vi "Query S Parameters.vi"(8 "error in (no error)":errorcluster, 10 "Sparameters (string)":string[](array[string]), 11 "VNA-ZNB in":refnum<class "VNA-ZNB.lvclass">) -> (0 "error out":errorcluster, 2 "S Parameters":T1[](array[typedef]), 3 "VNA-ZNB out":refnum<class "VNA-ZNB.lvclass">)   [LabVIEW 2020, in "VNA-ZNB.lvclass"]
doc: "Queryes the S parameter choosen. It can give single parameter or full 2 to 4 port parameters."
uses:
  VNA-ZNB.lvclass
  C:/Sandbox/Git_Sandbox/WiSpry Test Framework source code (LV20)/WiSpry Test Framework/Instruments/Instrument.lvclass
  C:/Sandbox/Git_Sandbox/WiSpry Test Framework source code (LV20)/WiSpry Test Framework/Instruments/Vector Network Analyzer/Vector Network Analyzer.lvclass
  Controls/Sparameter cluster.ctl
  Instrument.lvclass/Instrument.ctl
  Vector Network Analyzer.lvclass/Vector Network Analyzer.ctl
  Instrument.lvclass
  Vector Network Analyzer.lvclass
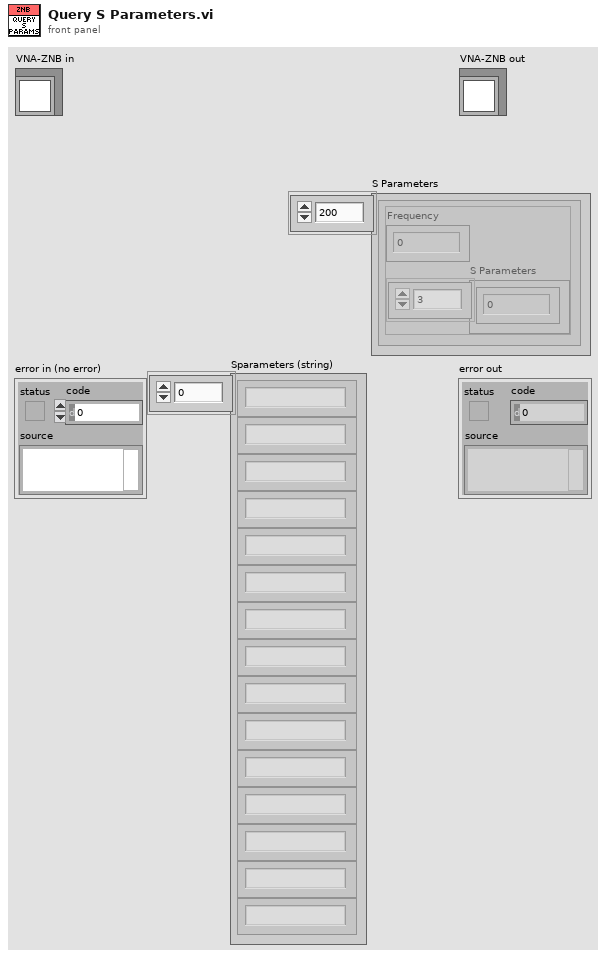
[diagram p1: front panel]
types:
  T1 = typedef "Vector Network Analyzer.lvclass/Sparameter cluster.ctl" = cluster{"Frequency":dbl, "S Parameters":cdb[]}
  T2 = enum16{"big-endian, network order", "native, host order", "little-endian"}
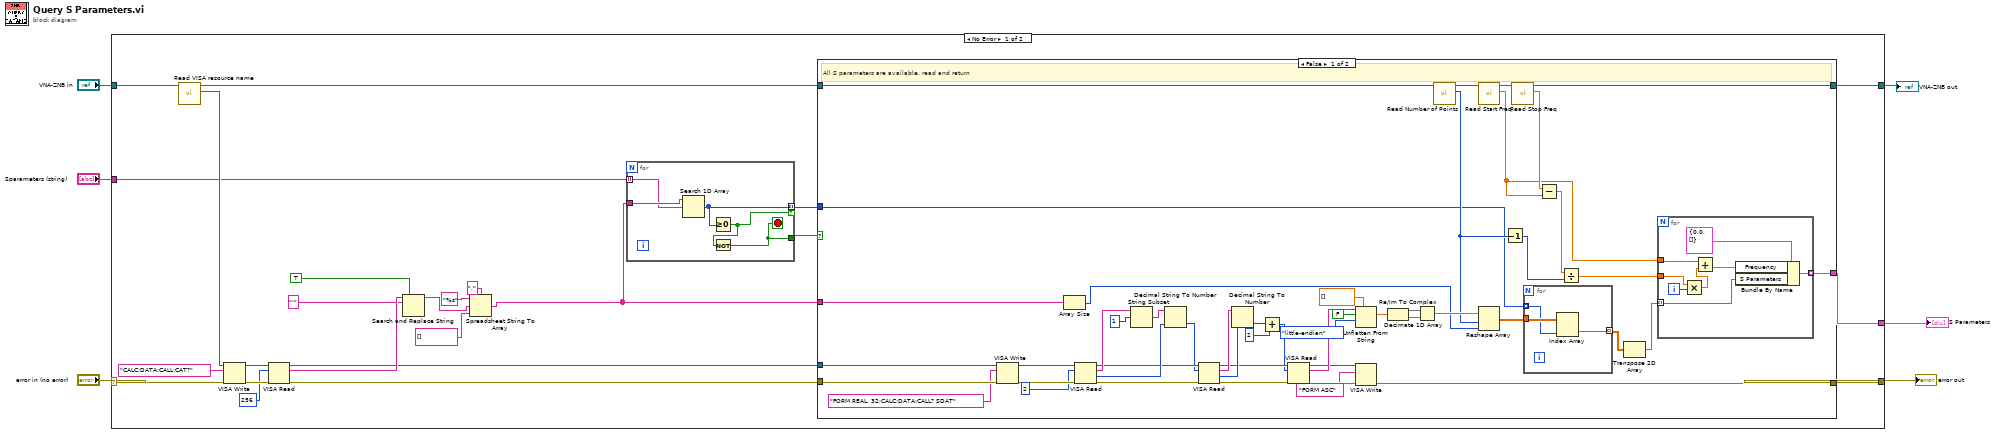
[diagram p0: block diagram]
diagram:
  n1 = case shown="No Error" "error in (no error)" {
    selector: "error in (no error)" -> [w29 w99]
    tunnel: "VNA-ZNB in" -> [w30 w98]
    tunnel: [w13 w98] -> w4
    tunnel: [w8 w99] -> w3
    tunnel: [w12 _] -> w2
    tunnel: "Sparameters (string)" -> [w7 _]
    frame No Error {
      n2 = call "Read VISA resource name.vi"("Instrument in"=w30) -> ("VISA resource name"=w28:refnum<visa-resource-name>, "Instrument out"=w14:refnum<class "VNA-ZNB.lvclass">)  [unwired: 9 in]
      n3 = VISA Write(VISA resource name=w28, write buffer="CALC:DATA:CALL:CAT?", error in (no error)=w29) -> (VISA resource name out=w25:refnum<visa-resource-name>, error out=w26:errorcluster)  [unwired: 1 out]
      n4 = VISA Read(VISA resource name=w25, byte count=u32 256, error in (no error)=w26) -> (VISA resource name out=w15:refnum<visa-resource-name>, read buffer=w23:string, error out=w16:errorcluster)  [unwired: 1 out]
      n5 = Search and Replace String(replace all?=TRUE ("replace all? (F)"), input string=w23, search string="'") -> (result string=w18:string)  [unwired: 5 in, 3 out]
      n6 = Spreadsheet String To Array(delimiter (Tab)=",", format string="%s", spreadsheet string=w18, array type (2D Dbl)=string[] []) -> (array=w11:string[])
      n7 = for {
        tunnel: w7 -> [w96] mode=indexing
        tunnel: w11 -> [w97]
        tunnel: [w95] -> w10 mode=indexing if=w94
        tunnel: [w93] -> w9
        stop <- w93 stop-if-true
        n8 = Search 1D Array(1D array=w97, element=w96) -> (index of element=w95:i32)  [unwired: 1 in]
        n9 = Greater Or Equal To 0?(x=w95) -> (x >= 0?=w94:bool)
        n10 = Not(x=w94) -> (.not. x?=w93:bool)
      }
      n11 = case shown="False" w9 {
        tunnel: w16 -> [w79 w92]
        tunnel: w15 -> [w78 _]
        tunnel: w14 -> [w51 w91]
        tunnel: [w45 w91] -> w13
        tunnel: [w44 _] -> w12
        tunnel: w11 -> [w39 _]
        tunnel: w10 -> [w37 _]
        tunnel: [w31 w92] -> w8
        frame False {
          # "All S parameters are available, read and return"
          n12 = VISA Write(VISA resource name=w78, write buffer="FORM REAL, 32;CALC:DATA:CALL? SDAT", error in (no error)=w79) -> (VISA resource name out=w75:refnum<visa-resource-name>, error out=w76:errorcluster)  [unwired: 1 out]
          n13 = Array Size(array=w39) -> (size(s)=w42:i32)
          n14 = VISA Read(VISA resource name=w75, byte count=u32 2, error in (no error)=w76) -> (VISA resource name out=w68:refnum<visa-resource-name>, read buffer=w71:string, return count=w70:u32, error out=w69:errorcluster)
          n15 = String Subset(string=w71, offset (0)=1) -> (substring=w72:string)  [unwired: 1 in]
          n16 = Decimal String To Number(string=w72, default (0L)=w70) -> (number=w67:u32)  [unwired: 1 in, 1 out]
          n17 = VISA Read(VISA resource name=w68, byte count=w67, error in (no error)=w69) -> (VISA resource name out=w62:refnum<visa-resource-name>, read buffer=w64:string, return count=w63:u32, error out=w60:errorcluster)
          n18 = Decimal String To Number(string=w64, default (0L)=w63) -> (number=w65:u32)  [unwired: 1 in, 1 out]
          n19 = Add(x=w65, y=u32 2) -> (x+y=w61:u32)
          n20 = VISA Read(VISA resource name=w62, byte count=w61, error in (no error)=w60) -> (VISA resource name out=w35:refnum<visa-resource-name>, read buffer=w59:string, error out=w36:errorcluster)  [unwired: 1 out]
          n21 = Unflatten From String(type=sgl[] [], binary string=w59, data includes array or string size? (T)=FALSE, byte order (0:big-endian, network order)=T2."little-endian") -> (value=w55:sgl[])  [unwired: 1 in, 2 out]
          n22 = VISA Write(VISA resource name=w35, write buffer="FORM ASC", error in (no error)=w36) -> (error out=w31:errorcluster)  [unwired: 2 out]
          n23 = Decimate 1D Array(w55) -> (w54:sgl[], w53:sgl[])
          n24 = Re/Im To Complex(1:w53, 2:w54) -> (0:w52:csg[])
          n25 = call "Read Number of Points.vi"("Vector Network Analyzer in"=w51) -> ("Number of Points"=w43:i32, "Vector Network Analyzer out"=w46:refnum<class "VNA-ZNB.lvclass">)  [unwired: 9 in]
          n26 = call "Read Start Freq.vi"("Vector Network Analyzer in"=w46) -> ("Start Freq"=w40:dbl, "Vector Network Analyzer out"=w47:refnum<class "VNA-ZNB.lvclass">)  [unwired: 9 in]
          n27 = Reshape Array(w52, w43, w42) -> (w38:csg[][])
          n28 = Decrement(x=w43) -> (x-1=w41:i32)
          n29 = call "Read Stop Freq.vi"("Vector Network Analyzer in"=w47) -> ("Stop Freq"=w48:dbl, "Vector Network Analyzer out"=w45:refnum<class "VNA-ZNB.lvclass">)  [unwired: 9 in]
          n30 = for {
            tunnel: w38 -> [w82]
            tunnel: w37 -> [w81] mode=indexing
            tunnel: [w80] -> w33 mode=indexing
            n31 = Index Array(array=w82, index (col)=w81) -> (element=w80:csg[])  [unwired: 1 in]
          }
          n32 = Subtract(x=w48, y=w40) -> (x-y=w49:dbl)
          n33 = Divide(x=w49, y=w41) -> (x/y=w50:dbl)
          n34 = Transpose 2D Array(2D array=w33) -> (transposed array=w32:csg[][])
          n35 = for {
            tunnel: w40 -> [w87]
            tunnel: w50 -> [w89]
            tunnel: [w84] -> w44 mode=indexing
            tunnel: w32 -> [w83] mode=indexing
            i -> [w90]
            n36 = Multiply(x=w89, y=w90) -> (x*y=w88:dbl)
            n37 = Add(x=w87, y=w88) -> (x+y=w85:dbl)
            n38 = Bundle By Name(cluster=T1 {"Frequency"=0.0, "S Parameters"=[]} ("S Parameters"), "Frequency"=w85, "S Parameters"=w83) -> (w84:T1)
          }
        }
        frame True {
          # "Add error handler"
          # "One of the parameters wanted is not available. Error"
        }
      }
    }
    frame Error {
    }
  }
  "error out" <- w3
  "VNA-ZNB out" <- w4
  "S Parameters" <- w2
